vi "Load State Machine.vi"   [LabVIEW 2013]
uses:
  typedefs/fg_typedef.ctl
  typedefs/State Machine/singleUseSubstate.ctl
  <vilib>/Rock Robotics/WPI/Solenoid/WPI_SolenoidValue.ctl
  typedefs/DevRef Type.ctl
  typedefs/State Machine/subStates.ctl
  <vilib>/Rock Robotics/WPI/Solenoid/WPI_SolenoidGetEnum.vi
panel:
  # "A State Machine to Handle Loading for Either High or Low Goal Shots"
types:
  T1 = typedef "fg_typedef.ctl" = enum16{"Get", "Set"}
  T2 = typedef "DevRef Type.ctl" = enum16{"Shooter Solenoid", "Latch Solenoid", "Right Up Sensor", "Right Down Sensor", "Hold Sensor", "Arm Encoder"}
  T3 = typedef "WPI_SolenoidValue.ctl" = enum16{"Off", "On", "Forward", "Reverse"}
  T4 = typedef "singleUseSubstate.ctl" = enum16{"null", "wait", "shift high", "shift low", "extend shooter", "retract shooter", "latch", "unlatch", "end"}
  T5 = typedef "subStates.ctl" = enum16{"null", "wait", "driver control", "auto", "manual override", "hold position", "rotate", "pickup", "pass", "recover pass", "load", "goto shoot", "shoot high goal", "shoot low goal", "cancel arm", "cancel shooter", "end", "test"}
  T6 = typedef "WPI_SolenoidDevRef.ctl" = cluster{"DevStatus":errorcluster, "Solenoid Module":T7, "Forward Solenoid Channel":T8, "Reverse Solenoid Channel":T8}
  T7 = typedef "FPGA_TypedefSolenoidModule.ctl" = enum16{"Solenoid Module 1", "Solenoid Module 2"}
  T8 = typedef "WPI_SolenoidChannel.ctl" = enum8{"Solenoid 1", "Solenoid 2", "Solenoid 3", "Solenoid 4", "Solenoid 5", "Solenoid 6", "Solenoid 7", "Solenoid 8", "Invalid"}
  T9 = typedef "WPI_DigitalInputDevRef.ctl" = cluster{"DevStatus":errorcluster, "DIO Channel":T10, "Digital Module":T11}
  T10 = typedef "FPGA_DIOChannel.ctl" = enum8{"DIO 1", "DIO 2", "DIO 3", "DIO 4", "DIO 5", "DIO 6", "DIO 7", "DIO 8", "DIO 9", "DIO 10", "DIO 11", "DIO 12", "DIO 13", "DIO 14", "Invalid"}
  T11 = typedef "FPGA_TypedefDigitalModule.ctl" = enum16{"Digital Module 1", "Digital Module 2"}
  T12 = typedef "WPI_EncoderDevRef.ctl" = cluster{"DevStatus":errorcluster, "EncoderIndex":T13, "CounterIndex":T14, "DistancePerCount":dbl, "Decoding Type":T15}
  T13 = typedef "FPGA_EncoderIdx.ctl" = enum8{"Enc 0", "Enc 1", "Enc 2", "Enc 3", "Invalid"}
  T14 = typedef "FPGA_CounterCtrSystemIndex.ctl" = enum8{"Ctr 0", "Ctr 1", "Ctr 2", "Ctr 3", "Ctr 4", "Ctr 5", "Ctr 6", "Ctr 7", "Invalid"}
  T15 = typedef "WPI_EncoderType.ctl" = enum16{"1x", "2x", "4x"}
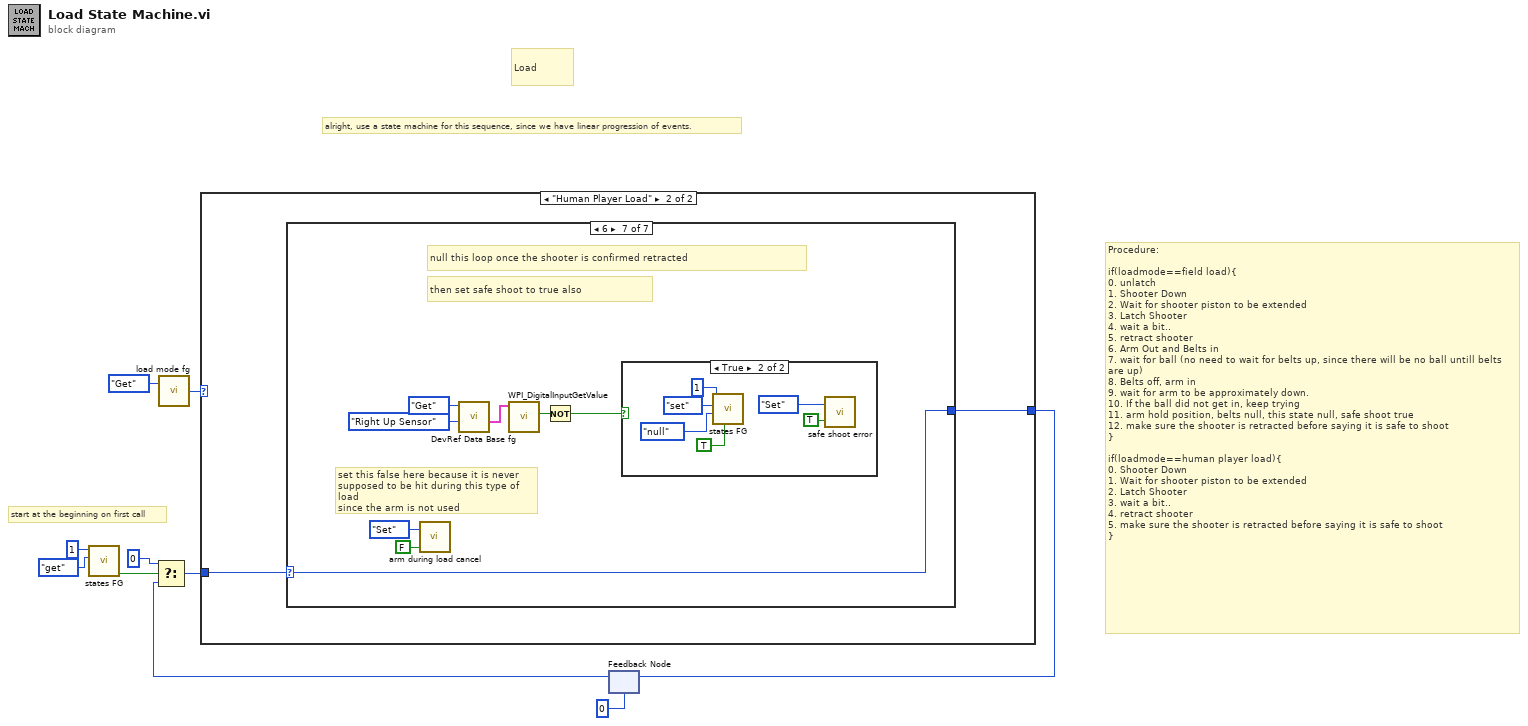
[diagram p0: block diagram]
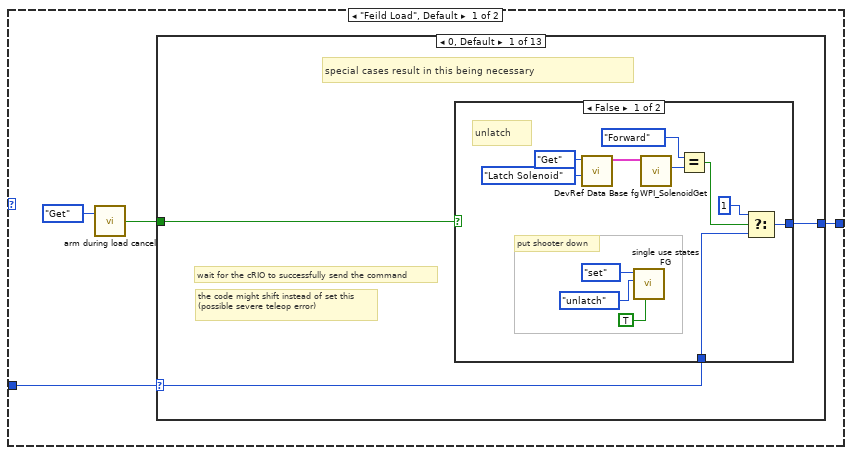
[diagram p2: hidden frame]
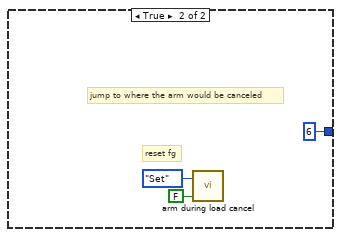
[diagram p3: hidden frame]
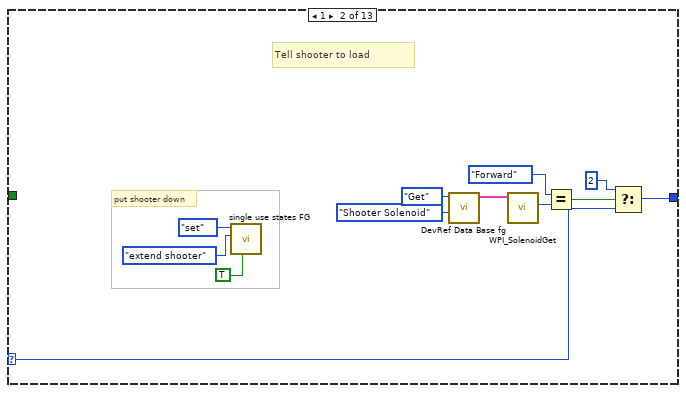
[diagram p4: hidden frame]
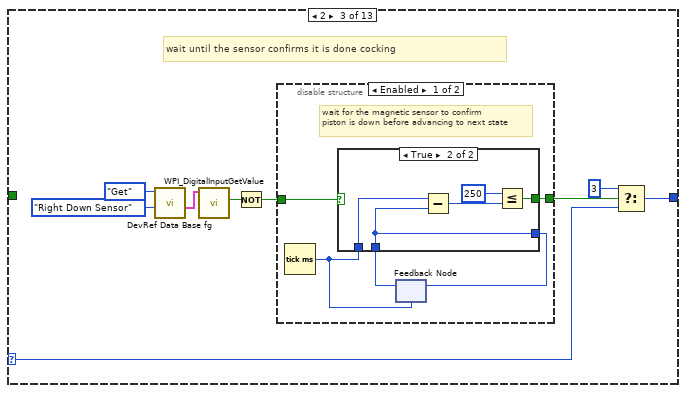
[diagram p5: hidden frame]
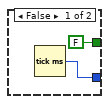
[diagram p6: hidden frame]
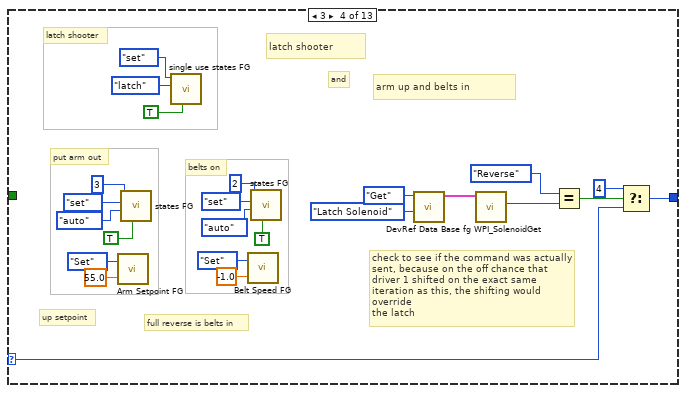
[diagram p8: hidden frame]
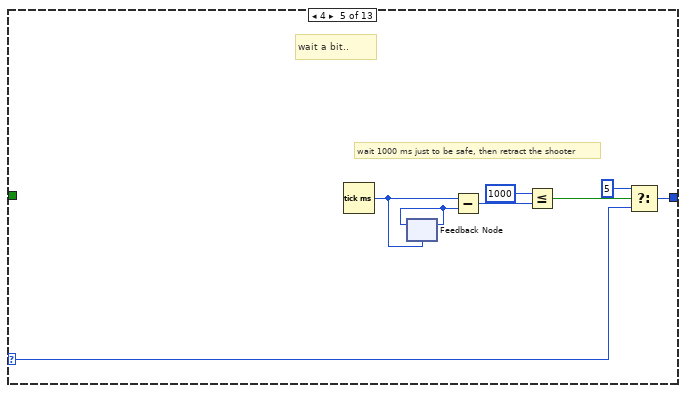
[diagram p9: hidden frame]
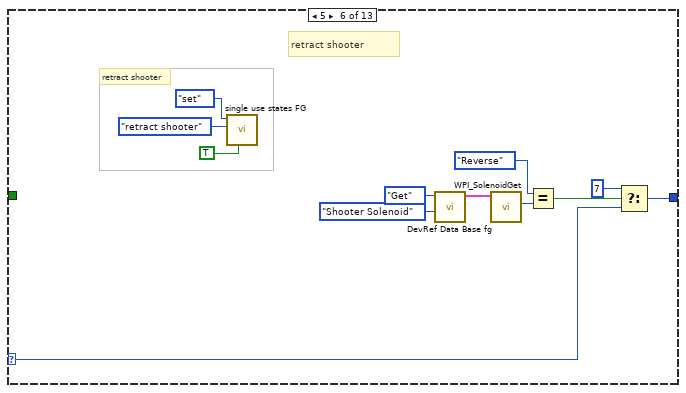
[diagram p10: hidden frame]
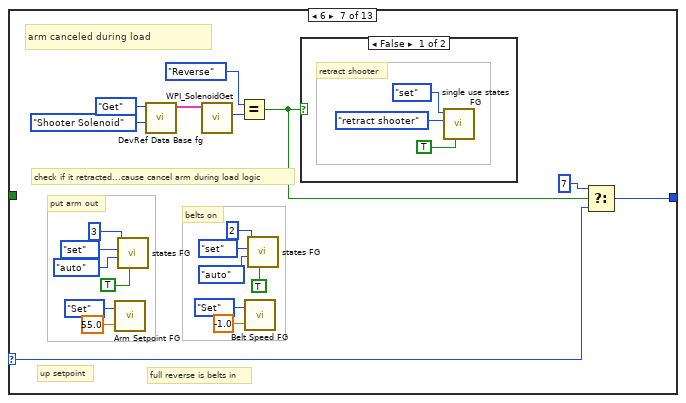
[diagram p11: hidden frame]
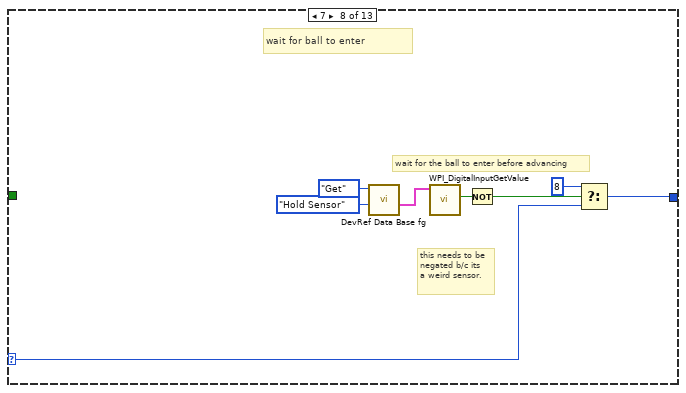
[diagram p13: hidden frame]
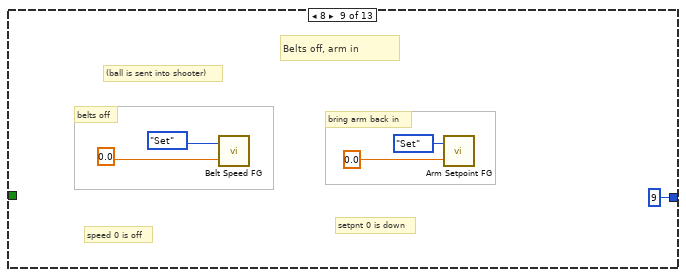
[diagram p14: hidden frame]
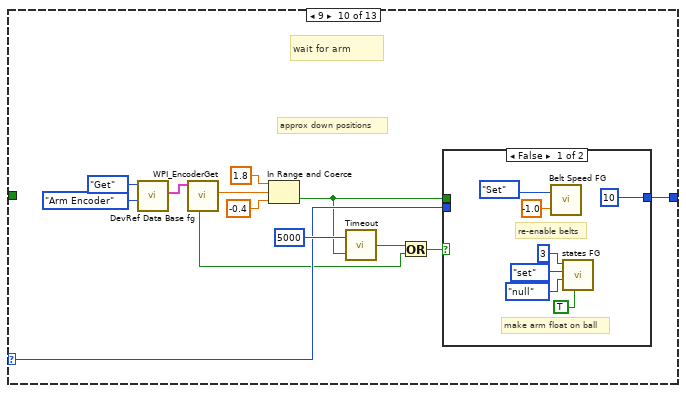
[diagram p15: hidden frame]
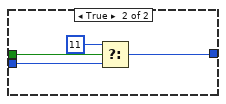
[diagram p16: hidden frame]
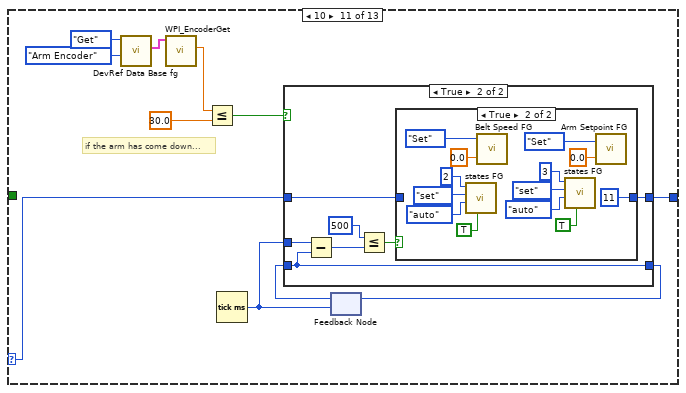
[diagram p17: hidden frame]
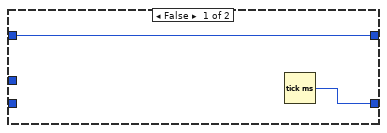
[diagram p18: hidden frame]
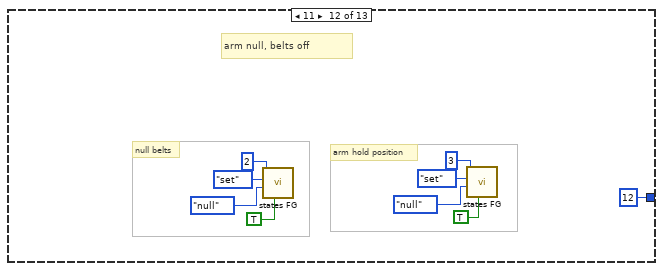
[diagram p20: hidden frame]
diagram:
  # "start at the beginning on first call"
  # "Load"
  # "Procedure: \n\nif(loadmode==field load){\n0. unlatch\n1. Shooter Down \n2. Wait for shooter piston to be extended\n3. Latch Shooter\n4. wait a bit..\n5. retract shooter\n6. Arm Out and Belts in\n7. wait for ball (no need to wait for belts up, since there will be no ball untill belts are up)\n8. Belts off, arm in\n9. wait for arm to be approximately down.\n10. If the ball did not get in, keep trying\n11. arm hold position, belts null, this state null, safe shoot true\n12. make sure the shooter is retracted before saying it is safe to shoot\n}\n\nif(loadmode==human player load){\n0. Shooter Down \n1. Wait for shooter piston to be extended\n2. Latch Shooter\n3. wait a bit..\n4. retract shooter\n5. make sure the shooter is retracted before saying it is safe to shoot\n}"
  # "alright, use a state machine for this sequence, since we have linear progression of events."
  n1 = call "states FG.vi"("menu (get)"=enum16{"set", "get"}."get", "Loop ID"=1) -> ("first call?"=w3:bool)  [unwired: 6 in, 3 out]
  n2 = call "load mode fg.vi"("Menu"=fg_typedef."Get") -> ("Load Mode"=w2:enum16{"Feild Load", "Human Player Load"})  [unwired: 1 in]
  n3 = feedback #1(u8 0) -> (w4:u8)
  n4 = Select(t=u8 0, s=w3, f=w4) -> (s? t:f=w6:u8)
  n5 = case shown="\"Human Player Load\"" w2 {
    tunnel: [w14 w228] -> w9
    tunnel: w6 -> [w13 w227]
    frame "Feild Load", Default {
      n6 = call "arm during load cancel.vi"("Mode"=enum16{"Get", "Set", "Teleop Set"}."Get") -> ("Arm Canceled During Load"=w11:bool)  [unwired: 1 in]
      n7 = case shown="0, Default" w13 {
        selector: w13 -> [w16 w33 w51 w86 w92 w110 w123 w140 _ w152 w172 _ w220]
        tunnel: [w17 w34 w50 w87 w94 w109 w124 w139 u8 9 ("t") w153 w174 u8 12 ("t") w220] -> w14
        tunnel: w11 -> [w15 _ _ _ _ _ _ _ _ _ _ _ _]
        frame 0, Default {
          # "the code might shift instead of set this\n(possible severe teleop error)"
          # "special cases result in this being necessary"
          # "wait for the cRIO to successfully send the command"
          n8 = case shown="False" w15 {
            tunnel: [w26 u8 6 ("t")] -> w17
            tunnel: w16 -> [w25 _]
            frame False {
              # "unlatch"
              # "put shooter down"
              n9 = call "DevRef Data Base fg.vi"("DevRef to Get"=DevRef_Type."Latch Solenoid", "Menu"=fg_typedef."Get") -> ("Selected Solenoid"=w24:T6)  [unwired: 1 in, 8 out]
              n10 = call "single use states FG.vi"("exit in"=TRUE, "substate"=singleUseSubstate."unlatch", "menu (get)"=enum16{"set", "get"}."set") -> ()  [unwired: 5 in, 4 out]
              n11 = call-poly <vilib>:"WPI_SolenoidGet.vi"("SolenoidDevRef"=w24) -> ("Value"=w23:T3)  [unwired: 8 in, 2 out]
              n12 = Equal?(x=WPI_SolenoidValue."Forward", y=w23) -> (x = y?=w21:bool)
              n13 = Select(t=u8 1, s=w21, f=w25) -> (s? t:f=w26:u8)
            }
            frame True {
              # "reset fg"
              # "jump to where the arm would be canceled"
              n14 = call "arm during load cancel.vi"("Arm Canceled During Load?"=FALSE, "Mode"=enum16{"Get", "Set", "Teleop Set"}."Set") -> ()  [unwired: 1 out]
            }
          }
        }
        frame 1 {
          # "Tell shooter to load"
          # "put shooter down"
          n15 = call "single use states FG.vi"("exit in"=TRUE, "substate"=singleUseSubstate."extend shooter", "menu (get)"=enum16{"set", "get"}."set") -> ()  [unwired: 5 in, 4 out]
          n16 = call "DevRef Data Base fg.vi"("DevRef to Get"=DevRef_Type."Shooter Solenoid", "Menu"=fg_typedef."Get") -> ("Selected Solenoid"=w41:T6)  [unwired: 1 in, 8 out]
          n17 = call-poly <vilib>:"WPI_SolenoidGet.vi"("SolenoidDevRef"=w41) -> ("Value"=w40:T3)  [unwired: 8 in, 2 out]
          n18 = Equal?(x=WPI_SolenoidValue."Forward", y=w40) -> (x = y?=w38:bool)
          n19 = Select(t=u8 2, s=w38, f=w33) -> (s? t:f=w34:u8)
        }
        frame 2 {
          # "wait until the sensor confirms it is done cocking"
          n20 = call "DevRef Data Base fg.vi"("DevRef to Get"=DevRef_Type."Right Down Sensor", "Menu"=fg_typedef."Get") -> ("Selected Sensor"=w52:T9)  [unwired: 1 in, 8 out]
          n21 = call <vilib>:"WPI_DigitalInputGetValue.vi"("DigitalInputDevRef"=w52) -> ("Value"=w53:bool)  [unwired: 8 in, 2 out]
          n22 = Not(x=w53) -> (.not. x?=w46:bool)
          n23 = disable-structure shown="Enabled" {
            disable-tunnel: w46 -> [w58 w66]
            disable-tunnel: [w54 w66] -> w45
            frame Enabled {
              # "wait for the magnetic sensor to confirm \npiston is down before advancing to next state"
              n24 = Tick Count (ms)() -> (millisecond timer value=w57:u32)
              n25 = feedback #2(w57) -> (w55:u32)
              n26 = case shown="True" w58 {
                tunnel: w57 -> [_ w63]
                tunnel: [w60 w61] -> w56
                tunnel: w55 -> [_ w61]
                tunnel: [FALSE w62] -> w54
                frame False {
                  n27 = Tick Count (ms)() -> (millisecond timer value=w60:u32)
                }
                frame True {
                  n28 = Subtract(x=w63, y=w61) -> (x-y=w65:u32)
                  n29 = Less Or Equal?(x=u32 250, y=w65) -> (x <= y?=w62:bool)
                }
              }
              n30 = feedback-in #2(w56) -> ()
            }
            frame Disabled {
            }
          }
          n31 = Select(t=u8 3, s=w45, f=w51) -> (s? t:f=w50:u8)
        }
        frame 3 {
          # "latch shooter"
          # "full reverse is belts in"
          # "belts on"
          # "up setpoint"
          # "put arm out"
          # "and"
          # "arm up and belts in"
          # "check to see if the command was actually\nsent, because on the off chance that\ndriver 1 shifted on the exact same\niteration as this, the shifting would override\nthe latch"
          # "latch shooter"
          n32 = call "Arm Setpoint FG.vi"("Setpoint In"=55.0, "Menu"=fg_typedef."Set") -> ()  [unwired: 1 out]
          n33 = call "states FG.vi"("exit in"=TRUE, "subState in"=subStates."auto", "menu (get)"=enum16{"set", "get"}."set", "Loop ID"=3) -> ()  [unwired: 4 in, 4 out]
          n34 = call "single use states FG.vi"("exit in"=TRUE, "substate"=singleUseSubstate."latch", "menu (get)"=enum16{"set", "get"}."set") -> ()  [unwired: 5 in, 4 out]
          n35 = call "Belt Speed FG.vi"("Speed In"=-1.0 ("Setpoint In"), "Menu"=fg_typedef."Set") -> ()  [unwired: 1 out]
          n36 = call "states FG.vi"("exit in"=TRUE, "subState in"=subStates."auto", "menu (get)"=enum16{"set", "get"}."set", "Loop ID"=2) -> ()  [unwired: 4 in, 4 out]
          n37 = call "DevRef Data Base fg.vi"("DevRef to Get"=DevRef_Type."Latch Solenoid", "Menu"=fg_typedef."Get") -> ("Selected Solenoid"=w85:T6)  [unwired: 1 in, 8 out]
          n38 = call-poly <vilib>:"WPI_SolenoidGet.vi"("SolenoidDevRef"=w85) -> ("Value"=w84:T3)  [unwired: 8 in, 2 out]
          n39 = Equal?(x=WPI_SolenoidValue."Reverse" ("Value"), y=w84) -> (x = y?=w82:bool)
          n40 = Select(t=u8 4, s=w82, f=w86) -> (s? t:f=w87:u8)
        }
        frame 4 {
          # "wait a bit.."
          # "wait 1000 ms just to be safe, then retract the shooter"
          n41 = Tick Count (ms)() -> (millisecond timer value=w96:u32)
          n42 = feedback #3(w96) -> (w97:u32)
          n43 = feedback-in #3(w97) -> ()
          n44 = Subtract(x=w96, y=w97) -> (x-y=w95:u32)
          n45 = Less Or Equal?(x=u32 1000, y=w95) -> (x <= y?=w93:bool)
          n46 = Select(t=u8 5, s=w93, f=w92) -> (s? t:f=w94:u8)
        }
        frame 5 {
          # "retract shooter"
          # "retract shooter"
          n47 = call "single use states FG.vi"("exit in"=TRUE, "substate"=singleUseSubstate."retract shooter", "menu (get)"=enum16{"set", "get"}."set") -> ()  [unwired: 5 in, 4 out]
          n48 = call "DevRef Data Base fg.vi"("DevRef to Get"=DevRef_Type."Shooter Solenoid", "Menu"=fg_typedef."Get") -> ("Selected Solenoid"=w108:T6)  [unwired: 1 in, 8 out]
          n49 = call-poly <vilib>:"WPI_SolenoidGet.vi"("SolenoidDevRef"=w108) -> ("Value"=w107:T3)  [unwired: 8 in, 2 out]
          n50 = Equal?(x=WPI_SolenoidValue."Reverse", y=w107) -> (x = y?=w105:bool)
          n51 = Select(t=u8 7, s=w105, f=w110) -> (s? t:f=w109:u8)
        }
        frame 6 {
          # "full reverse is belts in"
          # "belts on"
          # "up setpoint"
          # "put arm out"
          # "check if it retracted...cause cancel arm during load logic"
          # "arm canceled during load"
          n52 = call "Arm Setpoint FG.vi"("Setpoint In"=55.0, "Menu"=fg_typedef."Set") -> ()  [unwired: 1 out]
          n53 = call "states FG.vi"("exit in"=TRUE, "subState in"=subStates."auto", "menu (get)"=enum16{"set", "get"}."set", "Loop ID"=3) -> ()  [unwired: 4 in, 4 out]
          n54 = call "DevRef Data Base fg.vi"("DevRef to Get"=DevRef_Type."Shooter Solenoid", "Menu"=fg_typedef."Get") -> ("Selected Solenoid"=w131:T6)  [unwired: 1 in, 8 out]
          n55 = call-poly <vilib>:"WPI_SolenoidGet.vi"("SolenoidDevRef"=w131) -> ("Value"=w130:T3)  [unwired: 8 in, 2 out]
          n56 = Equal?(x=WPI_SolenoidValue."Reverse", y=w130) -> (x = y?=w125:bool)
          n57 = call "Belt Speed FG.vi"("Speed In"=-1.0 ("Setpoint In"), "Menu"=fg_typedef."Set") -> ()  [unwired: 1 out]
          n58 = call "states FG.vi"("exit in"=TRUE, "subState in"=subStates."auto", "menu (get)"=enum16{"set", "get"}."set", "Loop ID"=2) -> ()  [unwired: 4 in, 4 out]
          n59 = case shown="False" w125 {
            frame False {
              # "retract shooter"
              n60 = call "single use states FG.vi"("exit in"=TRUE, "substate"=singleUseSubstate."retract shooter", "menu (get)"=enum16{"set", "get"}."set") -> ()  [unwired: 5 in, 4 out]
            }
            frame True {
            }
          }
          n61 = Select(t=u8 7, s=w125, f=w123) -> (s? t:f=w124:u8)
        }
        frame 7 {
          # "this needs to be\nnegated b/c its\na weird sensor."
          # "wait for the ball to enter before advancing"
          # "wait for ball to enter"
          n62 = call "DevRef Data Base fg.vi"("DevRef to Get"=DevRef_Type."Hold Sensor", "Menu"=fg_typedef."Get") -> ("Selected Sensor"=w138:T9)  [unwired: 1 in, 8 out]
          n63 = call <vilib>:"WPI_DigitalInputGetValue.vi"("DigitalInputDevRef"=w138) -> ("Value"=w142:bool)  [unwired: 8 in, 2 out]
          n64 = Not(x=w142) -> (.not. x?=w141:bool)
          n65 = Select(t=u8 8, s=w141, f=w140) -> (s? t:f=w139:u8)
        }
        frame 8 {
          # "bring arm back in"
          # "setpnt 0 is down"
          # "speed 0 is off"
          # "Belts off, arm in"
          # "(ball is sent into shooter)"
          # "belts off"
          n66 = call "Belt Speed FG.vi"("Speed In"=0.0 ("Setpoint In"), "Menu"=fg_typedef."Set") -> ()  [unwired: 1 out]
          n67 = call "Arm Setpoint FG.vi"("Setpoint In"=0.0, "Menu"=fg_typedef."Set") -> ()  [unwired: 1 out]
        }
        frame 9 {
          # "approx down positions"
          # "wait for arm"
          n68 = call "DevRef Data Base fg.vi"("DevRef to Get"=DevRef_Type."Arm Encoder", "Menu"=fg_typedef."Get") -> ("Selected Encoder"=w160:T12)  [unwired: 1 in, 8 out]
          n69 = call <vilib>:"WPI_EncoderGet.vi"("EncoderDevRef"=w160) -> ("Distance"=w159:dbl, "Stopped"=w148:bool)  [unwired: 5 in, 4 out]
          n70 = In Range and Coerce(upper limit=1.8, x=w159, lower limit=-0.4) -> (In Range?=w151:bool)  [unwired: 1 out]
          n71 = call "Timeout.vi"("Done with Task?"=w151, "Timeout (ms)"=u32 5000) -> ("Timed Out?"=w149:bool)  [unwired: 1 in]
          n72 = Or(x=w149, y=w148) -> (x .or. y?=w150:bool)
          n73 = case shown="False" w150 {
            tunnel: w152 -> [_ w171]
            tunnel: [u8 10 ("t") w170] -> w153
            tunnel: w151 -> [_ w168]
            frame False {
              # "re-enable belts"
              # "make arm float on ball"
              n74 = call "Belt Speed FG.vi"("Speed In"=-1.0, "Menu"=fg_typedef."Set") -> ()  [unwired: 1 out]
              n75 = call "states FG.vi"("exit in"=TRUE, "subState in"=subStates."null", "menu (get)"=enum16{"set", "get"}."set", "Loop ID"=3) -> ()  [unwired: 4 in, 4 out]
            }
            frame True {
              n76 = Select(t=u8 11, s=w168, f=w171) -> (s? t:f=w170:u8)
            }
          }
        }
        frame 10 {
          # "if the arm has come down..."
          n77 = call "DevRef Data Base fg.vi"("DevRef to Get"=DevRef_Type."Arm Encoder", "Menu"=fg_typedef."Get") -> ("Selected Encoder"=w178:T12)  [unwired: 1 in, 8 out]
          n78 = call <vilib>:"WPI_EncoderGet.vi"("EncoderDevRef"=w178) -> ("Distance"=w182:dbl)  [unwired: 5 in, 5 out]
          n79 = Less Or Equal?(x=w182, y=30.0) -> (x <= y?=w173:bool)
          n80 = Tick Count (ms)() -> (millisecond timer value=w176:u32)
          n81 = feedback #4(w176) -> (w177:u32)
          n82 = case shown="True" w173 {
            tunnel: [w184 w191] -> w175
            tunnel: w177 -> [_ w191]
            tunnel: w176 -> [_ w190]
            tunnel: [w183 w186] -> w174
            tunnel: w172 -> [w183 w185]
            frame False {
              n83 = Tick Count (ms)() -> (millisecond timer value=w184:u32)
            }
            frame True {
              n84 = Subtract(x=w190, y=w191) -> (x-y=w189:u32)
              n85 = Less Or Equal?(x=u32 500, y=w189) -> (x <= y?=w187:bool)
              n86 = case shown="True" w187 {
                tunnel: [w192 u8 11] -> w186
                tunnel: w185 -> [w192 _]
                frame False {
                }
                frame True {
                  n87 = call "states FG.vi"("exit in"=TRUE, "subState in"=subStates."auto", "menu (get)"=enum16{"set", "get"}."set", "Loop ID"=2) -> ()  [unwired: 4 in, 4 out]
                  n88 = call "Belt Speed FG.vi"("Speed In"=0.0, "Menu"=fg_typedef."Set") -> ()  [unwired: 1 out]
                  n89 = call "states FG.vi"("exit in"=TRUE, "subState in"=subStates."auto", "menu (get)"=enum16{"set", "get"}."set", "Loop ID"=3) -> ()  [unwired: 4 in, 4 out]
                  n90 = call "Arm Setpoint FG.vi"("Setpoint In"=0.0, "Menu"=fg_typedef."Set") -> ()  [unwired: 1 out]
                }
              }
            }
          }
          n91 = feedback-in #4(w175) -> ()
        }
        frame 11 {
          # "null belts"
          # "arm null, belts off"
          # "arm hold position"
          n92 = call "states FG.vi"("exit in"=TRUE, "subState in"=subStates."null", "menu (get)"=enum16{"set", "get"}."set", "Loop ID"=2) -> ()  [unwired: 4 in, 4 out]
          n93 = call "states FG.vi"("exit in"=TRUE, "subState in"=subStates."null", "menu (get)"=enum16{"set", "get"}."set", "Loop ID"=3) -> ()  [unwired: 4 in, 4 out]
        }
        frame 12 {
          # "then set safe shoot to true also"
          # "null this loop once the shooter is confirmed retracted"
          n94 = call "DevRef Data Base fg.vi"("DevRef to Get"=DevRef_Type."Right Up Sensor", "Menu"=fg_typedef."Get") -> ("Selected Sensor"=w219:T9)  [unwired: 1 in, 8 out]
          n95 = call <vilib>:"WPI_DigitalInputGetValue.vi"("DigitalInputDevRef"=w219) -> ("Value"=w218:bool)  [unwired: 8 in, 2 out]
          n96 = Not(x=w218) -> (.not. x?=w217:bool)
          n97 = case shown="True" w217 {
            frame False {
            }
            frame True {
              n98 = call "states FG.vi"("exit in"=TRUE, "subState in"=subStates."null", "menu (get)"=enum16{"set", "get"}."set", "Loop ID"=1) -> ()  [unwired: 4 in, 4 out]
              n99 = call "safe shoot error.vi"("Can Shoot Safely?"=TRUE, "Menu"=fg_typedef."Set") -> ()  [unwired: 1 out]
            }
          }
        }
      }
    }
    frame "Human Player Load" {
      n100 = case shown="6" w227 {
        selector: w227 -> [w229 w251 w260 w282 w288 w303 w314]
        tunnel: [w230 w252 w259 w283 w290 w302 w314] -> w228
        frame 0, Default {
          # "put shooter down"
          # "since that has caused probelms not having this"
          # "unlatch"
          n101 = call "single use states FG.vi"("exit in"=TRUE, "substate"=singleUseSubstate."unlatch", "menu (get)"=enum16{"set", "get"}."set") -> ()  [unwired: 5 in, 4 out]
          n102 = call "DevRef Data Base fg.vi"("DevRef to Get"=DevRef_Type."Latch Solenoid", "Menu"=fg_typedef."Get") -> ("Selected Solenoid"=w237:T6)  [unwired: 1 in, 8 out]
          n103 = call-poly <vilib>:"WPI_SolenoidGet.vi"("SolenoidDevRef"=w237) -> ("Value"=w236:T3)  [unwired: 8 in, 2 out]
          n104 = Equal?(x=WPI_SolenoidValue."Forward", y=w236) -> (x = y?=w234:bool)
          n105 = Select(t=u8 1, s=w234, f=w229) -> (s? t:f=w230:u8)
        }
        frame 1 {
          # "put shooter down"
          # "Wait for shooter to be cocked"
          # "Tell shooter to load"
          n106 = call "single use states FG.vi"("exit in"=TRUE, "substate"=singleUseSubstate."extend shooter", "menu (get)"=enum16{"set", "get"}."set") -> ()  [unwired: 5 in, 4 out]
          n107 = call "DevRef Data Base fg.vi"("DevRef to Get"=DevRef_Type."Shooter Solenoid", "Menu"=fg_typedef."Get") -> ("Selected Solenoid"=w247:T6)  [unwired: 1 in, 8 out]
          n108 = call-poly <vilib>:"WPI_SolenoidGet.vi"("SolenoidDevRef"=w247) -> ("Value"=w246:T3)  [unwired: 8 in, 2 out]
          n109 = Equal?(x=WPI_SolenoidValue."Forward", y=w246) -> (x = y?=w244:bool)
          n110 = Select(t=u8 2, s=w244, f=w251) -> (s? t:f=w252:u8)
        }
        frame 2 {
          # "wait for the magnetic sensor to confirm \npiston is down before advancing to next state"
          # "wait until the sensor confirms it is done cocking"
          n111 = call "DevRef Data Base fg.vi"("DevRef to Get"=DevRef_Type."Right Down Sensor", "Menu"=fg_typedef."Get") -> ("Selected Sensor"=w261:T9)  [unwired: 1 in, 8 out]
          n112 = call <vilib>:"WPI_DigitalInputGetValue.vi"("DigitalInputDevRef"=w261) -> ("Value"=w254:bool)  [unwired: 8 in, 2 out]
          n113 = Not(x=w254) -> (.not. x?=w255:bool)
          n114 = disable-structure shown="Enabled" {
            disable-tunnel: w255 -> [w266 w274]
            disable-tunnel: [w262 w274] -> w253
            frame Enabled {
              n115 = Tick Count (ms)() -> (millisecond timer value=w265:u32)
              n116 = feedback #5(w265) -> (w263:u32)
              n117 = case shown="True" w266 {
                tunnel: w265 -> [_ w271]
                tunnel: [w268 w269] -> w264
                tunnel: w263 -> [_ w269]
                tunnel: [FALSE w270] -> w262
                frame False {
                  n118 = Tick Count (ms)() -> (millisecond timer value=w268:u32)
                }
                frame True {
                  n119 = Subtract(x=w271, y=w269) -> (x-y=w273:u32)
                  n120 = Less Or Equal?(x=u32 250, y=w273) -> (x <= y?=w270:bool)
                }
              }
              n121 = feedback-in #5(w264) -> ()
            }
            frame Disabled {
            }
          }
          n122 = Select(t=u8 3, s=w253, f=w260) -> (s? t:f=w259:u8)
        }
        frame 3 {
          # "latch shooter"
          # "check to see if the command was actually\nsent, because on the off chance that\ndriver 1 shifted on the exact same\niteration as this, the shifting would override\nthe latch (applies to all instances of this type\nof code logic)"
          # "latch shooter"
          n123 = call "single use states FG.vi"("exit in"=TRUE, "substate"=singleUseSubstate."latch", "menu (get)"=enum16{"set", "get"}."set") -> ()  [unwired: 5 in, 4 out]
          n124 = call "DevRef Data Base fg.vi"("DevRef to Get"=DevRef_Type."Latch Solenoid", "Menu"=fg_typedef."Get") -> ("Selected Solenoid"=w281:T6)  [unwired: 1 in, 8 out]
          n125 = call-poly <vilib>:"WPI_SolenoidGet.vi"("SolenoidDevRef"=w281) -> ("Value"=w280:T3)  [unwired: 8 in, 2 out]
          n126 = Equal?(x=WPI_SolenoidValue."Reverse" ("Value"), y=w280) -> (x = y?=w278:bool)
          n127 = Select(t=u8 4, s=w278, f=w282) -> (s? t:f=w283:u8)
        }
        frame 4 {
          # "wait a bit.."
          # "wait 1000 ms just to be safe, then retract the shooter"
          n128 = Tick Count (ms)() -> (millisecond timer value=w292:u32)
          n129 = feedback #6(w292) -> (w293:u32)
          n130 = feedback-in #6(w293) -> ()
          n131 = Subtract(x=w292, y=w293) -> (x-y=w291:u32)
          n132 = Less Or Equal?(x=u32 1000, y=w291) -> (x <= y?=w289:bool)
          n133 = Select(t=u8 5, s=w289, f=w288) -> (s? t:f=w290:u8)
        }
        frame 5 {
          # "retract shooter"
          # "retract shooter"
          n134 = call "single use states FG.vi"("exit in"=TRUE, "substate"=singleUseSubstate."retract shooter", "menu (get)"=enum16{"set", "get"}."set") -> ()  [unwired: 5 in, 4 out]
          n135 = call "DevRef Data Base fg.vi"("DevRef to Get"=DevRef_Type."Shooter Solenoid", "Menu"=fg_typedef."Get") -> ("Selected Solenoid"=w301:T6)  [unwired: 1 in, 8 out]
          n136 = call-poly <vilib>:"WPI_SolenoidGet.vi"("SolenoidDevRef"=w301) -> ("Value"=w300:T3)  [unwired: 8 in, 2 out]
          n137 = Equal?(x=WPI_SolenoidValue."Reverse", y=w300) -> (x = y?=w298:bool)
          n138 = Select(t=u8 6, s=w298, f=w303) -> (s? t:f=w302:u8)
        }
        frame 6 {
          # "set this false here because it is never\nsupposed to be hit during this type of load\nsince the arm is not used"
          # "then set safe shoot to true also"
          # "null this loop once the shooter is confirmed retracted"
          n139 = call "arm during load cancel.vi"("Arm Canceled During Load?"=FALSE, "Mode"=enum16{"Get", "Set", "Teleop Set"}."Set") -> ()  [unwired: 1 out]
          n140 = call "DevRef Data Base fg.vi"("DevRef to Get"=DevRef_Type."Right Up Sensor", "Menu"=fg_typedef."Get") -> ("Selected Sensor"=w313:T9)  [unwired: 1 in, 8 out]
          n141 = call <vilib>:"WPI_DigitalInputGetValue.vi"("DigitalInputDevRef"=w313) -> ("Value"=w312:bool)  [unwired: 8 in, 2 out]
          n142 = Not(x=w312) -> (.not. x?=w311:bool)
          n143 = case shown="True" w311 {
            frame False {
            }
            frame True {
              n144 = call "states FG.vi"("exit in"=TRUE, "subState in"=subStates."null", "menu (get)"=enum16{"set", "get"}."set", "Loop ID"=1) -> ()  [unwired: 4 in, 4 out]
              n145 = call "safe shoot error.vi"("Can Shoot Safely?"=TRUE, "Menu"=fg_typedef."Set") -> ()  [unwired: 1 out]
            }
          }
        }
      }
    }
  }
  n146 = feedback-in #1(w9) -> ()
